vi "Plot GetModifiers.vi"(11 "Start String":string) -> (0 "Error":bool, 1 "Precision":i32, 2 "Code Character":string, 3 "Remaining String":string, 4 "Min Width":u16, 5 "Modifiers":string)   [LabVIEW 2017, in "3D Plot.lvclass"]
uses:
  <vilib>/Math Plots/3D Math Plots/3D Plot/3D Plot/3D Plot.lvclass
panel:
  out "*(type *) &x":u8[](array[numeric])
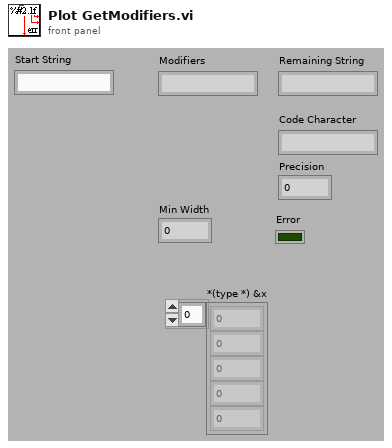
[diagram p1: front panel]
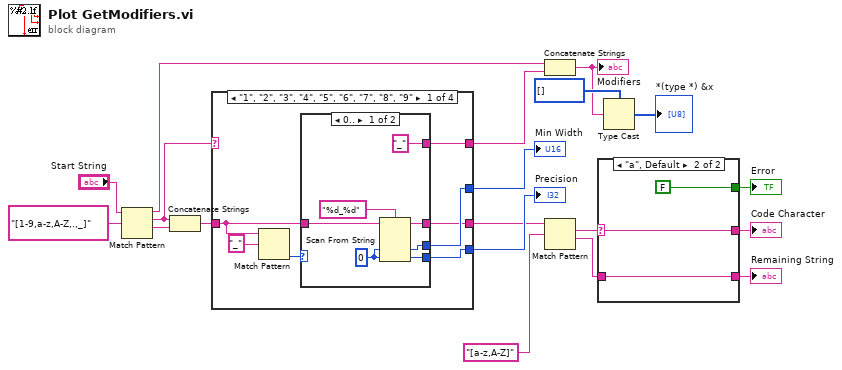
[diagram p0: block diagram]
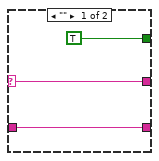
[diagram p2: hidden frame]
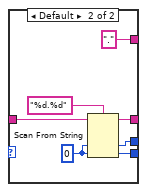
[diagram p3: hidden frame]
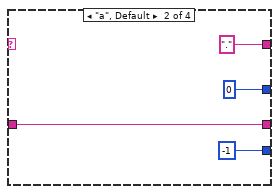
[diagram p4: hidden frame]
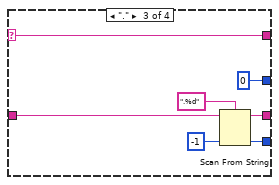
[diagram p5: hidden frame]
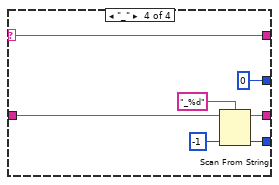
[diagram p6: hidden frame]
diagram:
  n1 = Match Pattern(string="Start String", regular expression="[1-9,a-z,A-Z,.,_]") -> (before substring=w2:string, match substring=w13:string, after substring=w17:string)  [unwired: 2 out]
  n2 = Concatenate Strings(w13, w17) -> (w16:string)
  n3 = case shown="\"1\", \"2\", \"3\", \"4\", \"5\", \"6\", \"7\", \"8\", \"9\"" w13 {
    selector: w13 -> [_ _ w45 w52]
    tunnel: w16 -> [w23 w44 w51 w58]
    tunnel: [w26 -1 ("default value 1") w47 w54] -> w15
    tunnel: [w25 0 ("default value 1") 0 ("default value 1") 0 ("default value 1")] -> w14
    tunnel: [w24 w44 w49 w56] -> w6
    tunnel: [w20 "." w45 w52] -> w3
    frame "1", "2", "3", "4", "5", "6", "7", "8", "9" {
      n4 = Match Pattern(string=w23, regular expression="_") -> (offset past match=w21:i32)  [unwired: 4 out]
      n5 = case shown="0.." w21 {
        tunnel: [w29 w38] -> w26
        tunnel: [w30 w37] -> w25
        tunnel: [w31 w36] -> w24
        tunnel: w23 -> [w28 w35]
        tunnel: ["_" "."] -> w20
        frame 0.. {
          w32 = 0 ("default value 1")
          n6 = Scan From String(format string="%d_%d", input string=w28, default 1=w32, default 2=w32) -> (remaining string=w31:string, output 1=w30:i32, output 2=w29:i32)  [unwired: 2 in, 2 out]
        }
        frame Default {
          w39 = 0 ("default value 1")
          n7 = Scan From String(format string="%d.%d", input string=w35, default 1=w39, default 2=w39) -> (remaining string=w36:string, output 1=w37:i32, output 2=w38:i32)  [unwired: 2 in, 2 out]
        }
      }
    }
    frame "a", Default {
    }
    frame "." {
      n8 = Scan From String(format string=".%d", input string=w51, default 1=-1 ("default value 1")) -> (remaining string=w49:string, output 1=w47:i32)  [unwired: 2 in, 2 out]
    }
    frame "_" {
      n9 = Scan From String(format string="_%d", input string=w58, default 1=-1 ("default value 1")) -> (remaining string=w56:string, output 1=w54:i32)  [unwired: 2 in, 2 out]
    }
  }
  "Min Width" <- w14
  "Precision" <- w15
  n10 = Concatenate Strings(w2, w3) -> (w1:string)
  "Modifiers" <- w1
  n11 = Match Pattern(string=w6, regular expression="[a-z,A-Z]") -> (match substring=w11:string, after substring=w7:string)  [unwired: 3 out]
  n12 = case shown="\"a\", Default" w11 {
    selector: w11 -> [w60 w64]
    tunnel: [TRUE FALSE] -> w10
    tunnel: [w60 w64] -> w9
    tunnel: [w59 w63] -> w8
    tunnel: w7 -> [w59 w63]
    frame "" {
    }
    frame "a", Default {
    }
  }
  "Code Character" <- w9
  "Remaining String" <- w8
  "Error" <- w10
  n13 = Type Cast(type=u8[] [], x=w1) -> (*(type *) &x=→"*(type *) &x":u8[])
